vi "17mart .vi"() -> ()   [LabVIEW 2020]
panel:
  out "array w/ subset deleted":i32[](array[numeric])
  out "Array 6":i32[](array[numeric])
  out "x+y 2":dbl[](array[numeric])
  out "output array":dbl[](array[numeric])
  in  "element 5":dbl
  out "subarray":dbl[](array[numeric])
  out "index teki yazan":dbl
  out "appended array":dbl[](array[numeric])
  out "initialized array 2":dbl[](array[numeric])
  in  "element 4":dbl
  in  "element 3":dbl
  out "x+y":dbl[][](array[numeric])
  in  "element 2":dbl
  out "initialized array":dbl[][](array[numeric])
  in  "element":dbl
  out "size(s) 2":i32[](array[numeric])
  out "Array 5":dbl[][](array[numeric])
  out "size(s)":i32
  out "i":i32[](array[numeric])
  in  "Array 4":dbl[](array[numeric])
  out "Array 3":dbl[](array[numeric])
  out "Array 2":dbl[](array[numeric])
  out "Array":dbl[][](array[numeric])
  in  "Numeric 2":i32
  in  "Numeric":i32
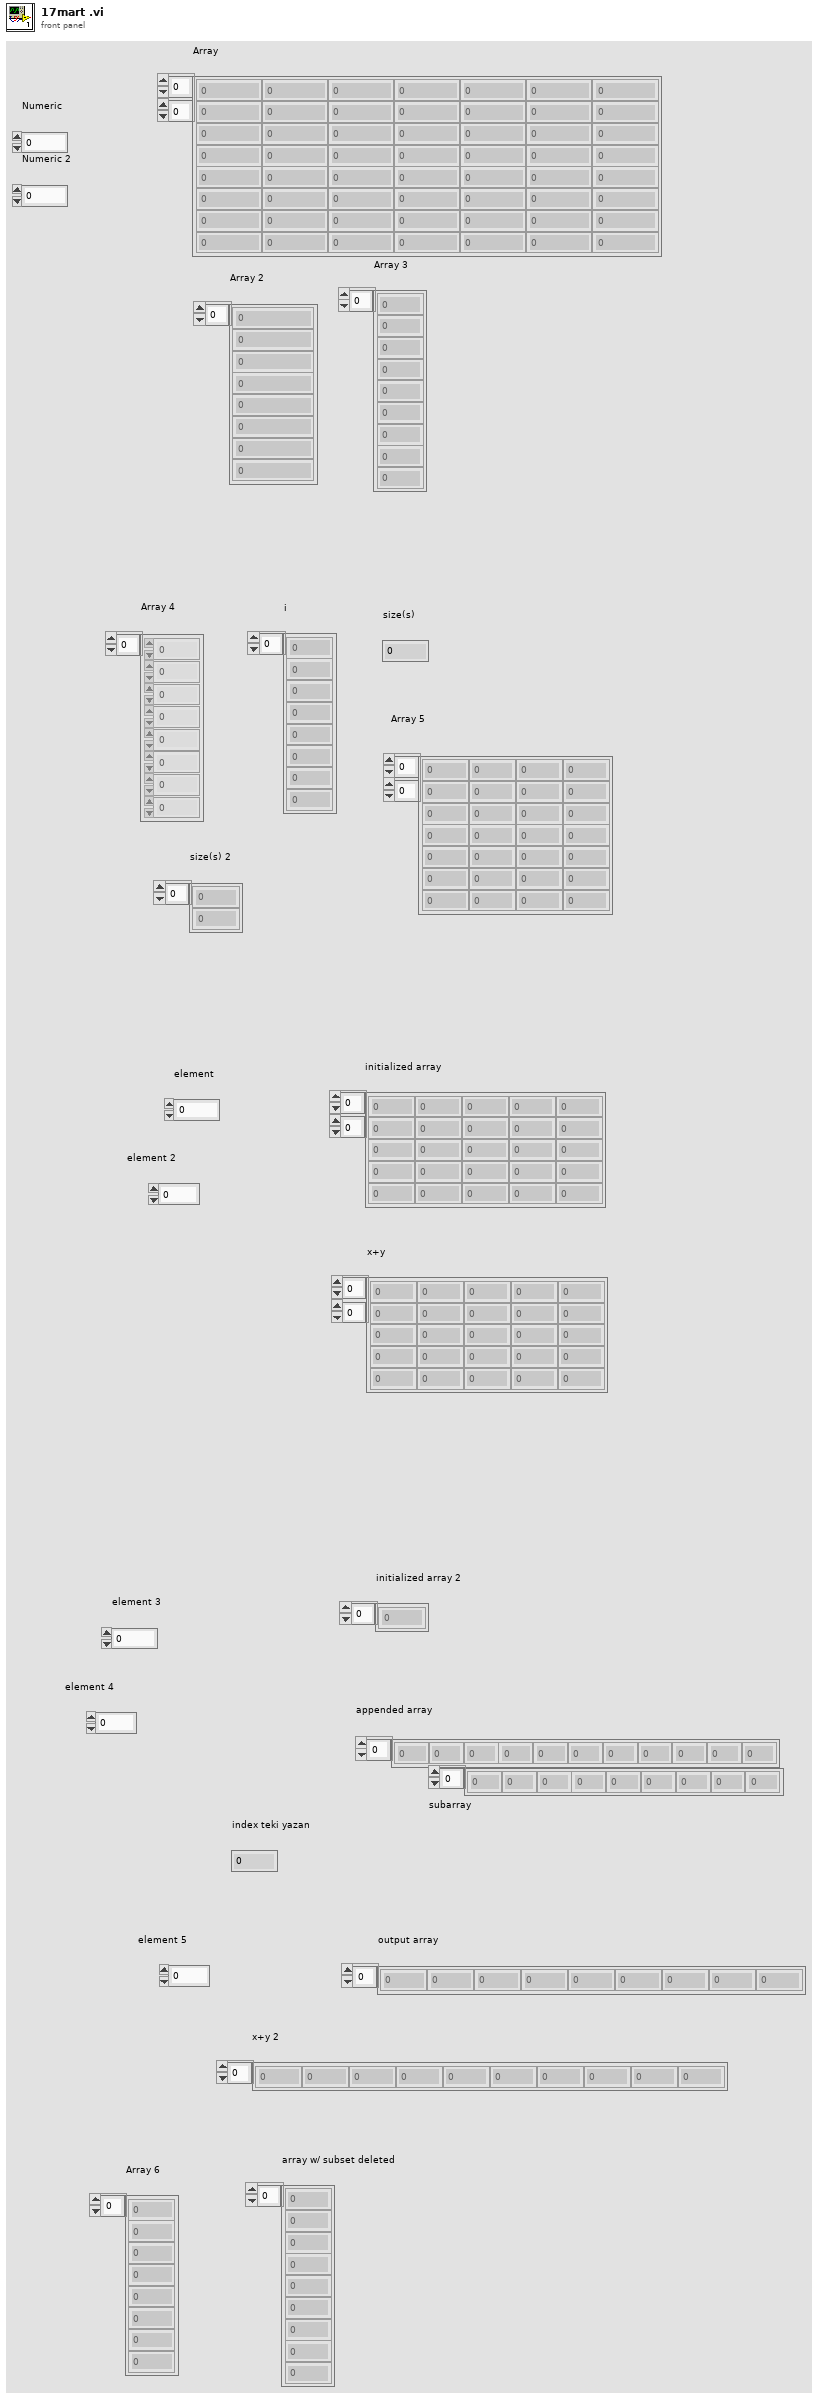
[diagram p1: front panel]
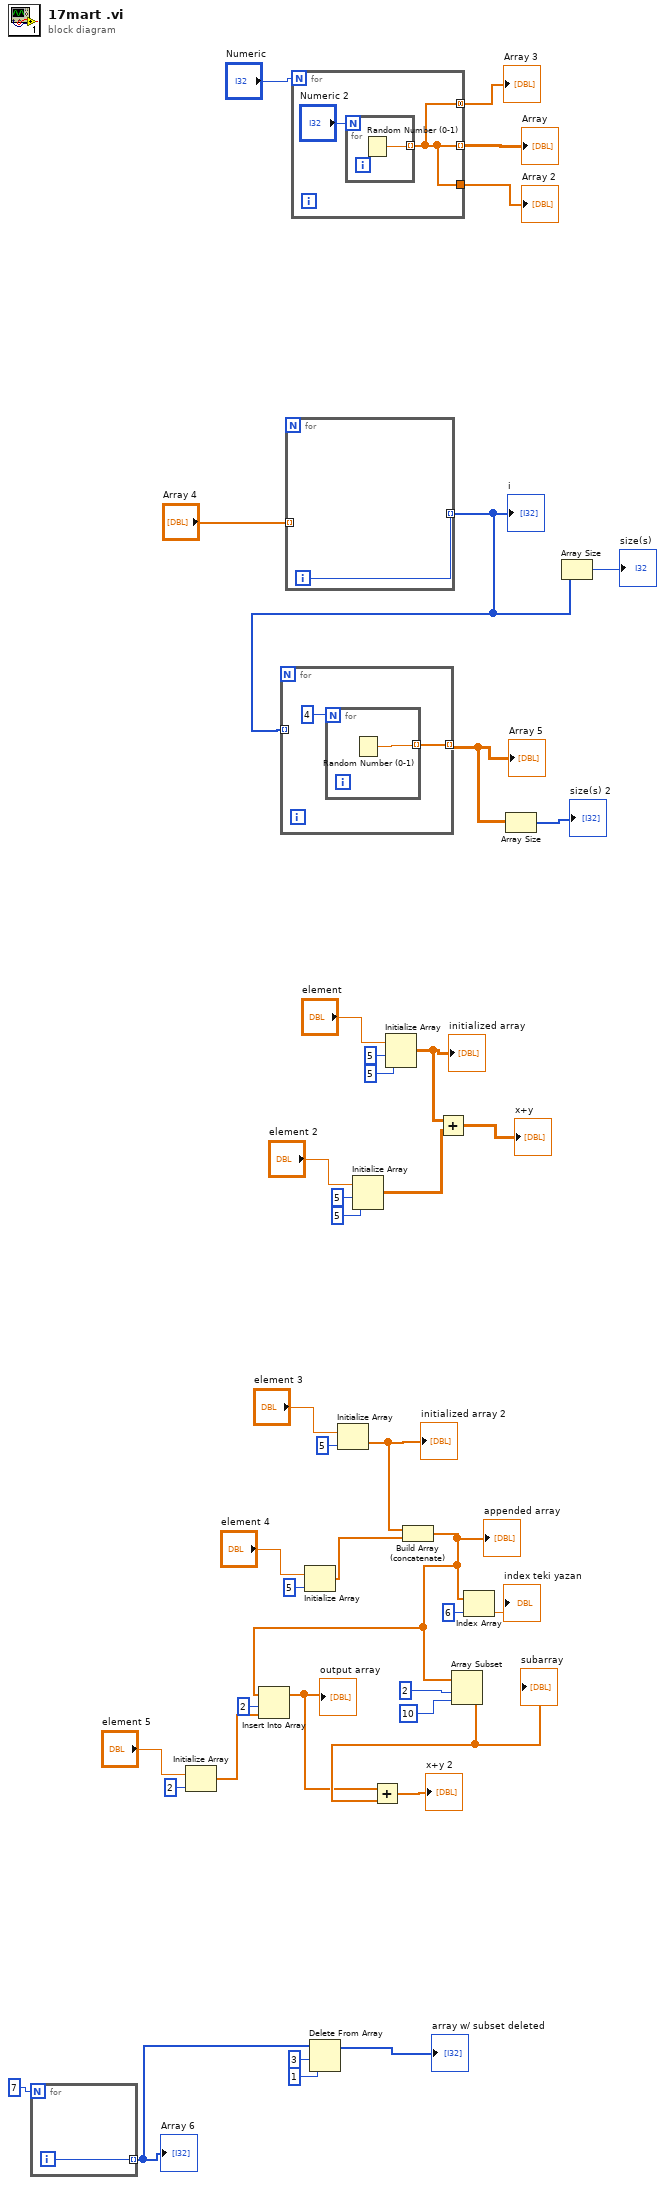
[diagram p0: block diagram]
diagram:
  n1 = for {
    N: 7 -> [_]
    tunnel: [w42] -> w2 mode=indexing
    i -> [w42]
  }
  "Array 6" <- w2
  n2 = Initialize Array("element 5", 2 ("dimension size")) -> (w10:dbl[])
  n3 = for {
    tunnel: "Array 4" -> [_] mode=indexing
    tunnel: [w43] -> w35 mode=indexing
    i -> [w43]
  }
  "i" <- w35
  n4 = for {
    tunnel: w35 -> [_] mode=indexing
    tunnel: [w44] -> w34 mode=indexing
    n5 = for {
      N: 4 -> [_]
      tunnel: [w46] -> w44 mode=indexing
      n6 = Random Number (0-1)() -> (number: 0 to 1=w46:dbl)
    }
  }
  "Array 5" <- w34
  n7 = for {
    N: "Numeric" -> [_]
    tunnel: [w47] -> w40 mode=indexing
    tunnel: [w47] -> w39
    tunnel: [w47] -> w38 mode=concatenating
    n8 = for {
      N: "Numeric 2" -> [_]
      tunnel: [w49] -> w47 mode=indexing
      n9 = Random Number (0-1)() -> (number: 0 to 1=w49:dbl)
    }
  }
  "Array" <- w40
  "Array 2" <- w39
  "Array 3" <- w38
  n10 = Initialize Array("element 4", 5 ("dimension size")) -> (w19:dbl[])
  n11 = Delete From Array(array=w2, length=3, index=1) -> (array with subset deleted=→"array w/ subset deleted":i32[])  [unwired: 1 out]
  n12 = Initialize Array("element 3", 5 ("dimension size")) -> (w18:dbl[])
  "initialized array 2" <- w18
  n13 = Initialize Array("element 2", 5 ("dimension size"), 5 ("dimension size")) -> (w25:dbl[][])
  n14 = Initialize Array("element", 5 ("dimension size"), 5 ("dimension size")) -> (w26:dbl[][])
  "initialized array" <- w26
  n15 = Build Array (concatenate)(w18, w19) -> (w9:dbl[])
  "appended array" <- w9
  n16 = Insert Into Array(array=w9, index=2, new element=w10) -> (w7:dbl[])
  "output array" <- w7
  n17 = Add(x=w26, y=w25) -> (x+y=→"x+y":dbl[][])
  n18 = Array Subset(array=w9, index=2, length=10) -> (w8:dbl[])
  "subarray" <- w8
  n19 = Add(x=w7, y=w8) -> (x+y=→"x+y 2":dbl[])
  n20 = Index Array(array=w9, index=6) -> (element=→"index teki yazan":dbl)
  n21 = Array Size(array=w34) -> (size(s)=→"size(s) 2":i32[])
  n22 = Array Size(array=w35) -> (size(s)=→"size(s)":i32)
